vi "Inicializacion_LoRa.vi"(11 "Inicializacion LoRa":T1={"Enviar direccion"=FALSE, "Direccion"=1} {"Direccion" min=1 max=127 step=1}) -> (2 "Enviar direccion":bool, 3 "Direccion":i16)   [LabVIEW 2022 SP3]
panel:
  # "Direccion fisiografo (1-127)"
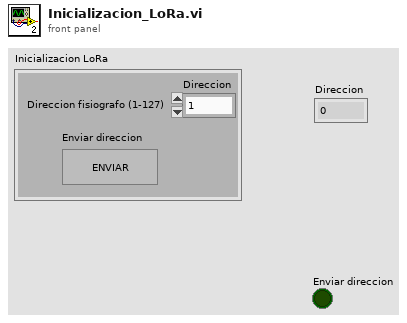
[diagram p1: front panel]
types:
  T1 = cluster{"Enviar direccion":bool, "Direccion":i16}
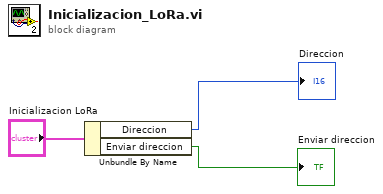
[diagram p0: block diagram]
diagram:
  n1 = Unbundle By Name("Inicializacion LoRa") -> ("Direccion"=→"Direccion":i16, "Enviar direccion"=→"Enviar direccion":bool)
